vi "Bool array to color.vi"(8 "error in (no error)":errorcluster, 11 "LED Panel":T2) -> (0 "error out":errorcluster, 3 "Calib color":T1)   [LabVIEW 2020]
uses:
  Controls/LED panel ---typedef.ctl
  Controls/Calibration color ---typedef.ctl
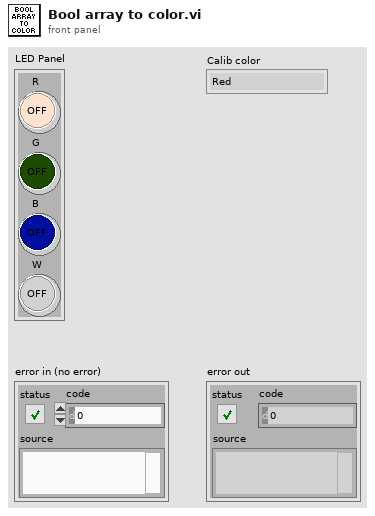
[diagram p1: front panel]
types:
  T1 = typedef "Calibration color ---typedef.ctl" = enum16{"Red", "Green", "Blue", "White", "All", "Reset", "Get"}
  T2 = typedef "LED panel ---typedef.ctl" = cluster{"R":bool, "G":bool, "B":bool, "W":bool}
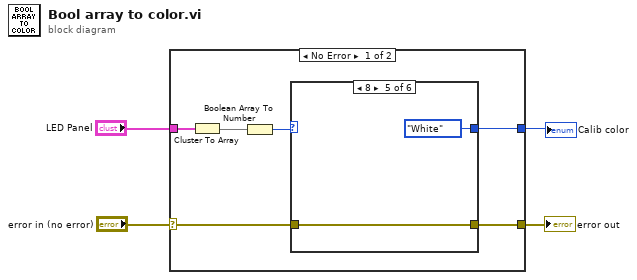
[diagram p0: block diagram]
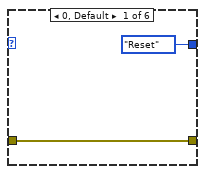
[diagram p2: hidden frame]
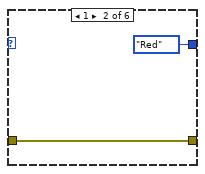
[diagram p3: hidden frame]
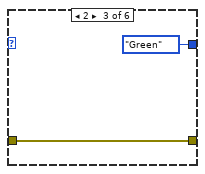
[diagram p4: hidden frame]
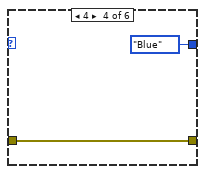
[diagram p5: hidden frame]
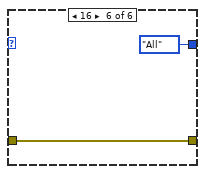
[diagram p6: hidden frame]
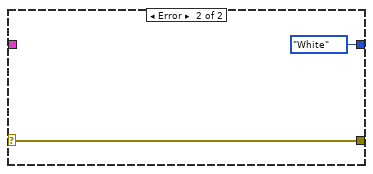
[diagram p7: hidden frame]
diagram:
  n1 = case shown="No Error" "error in (no error)" {
    selector: "error in (no error)" -> [w10 w24]
    tunnel: [w9 w24] -> w3
    tunnel: "LED Panel" -> [w8 _]
    tunnel: [w5 Calibration_color_---typedef."White" ("Calib color")] -> w1
    frame No Error {
      n2 = Cluster To Array(cluster=w8) -> (array=w6:bool[])
      n3 = Boolean Array To Number(Boolean array=w6) -> (number=w7:u32)
      n4 = case shown="8" w7 {
        tunnel: w10 -> [w12 w14 w16 w18 w20 w22]
        tunnel: [w12 w14 w16 w18 w20 w22] -> w9
        tunnel: [Calibration_color_---typedef."Reset" ("Calib color") Calibration_color_---typedef."Red" ("Calib color") Calibration_color_---typedef."Green" ("Calib color") Calibration_color_---typedef."Blue" ("Calib color") Calibration_color_---typedef."White" ("Calib color") Calibration_color_---typedef."All" ("Calib color")] -> w5
        frame 0, Default {
        }
        frame 1 {
        }
        frame 2 {
        }
        frame 4 {
        }
        frame 8 {
        }
        frame 16 {
        }
      }
    }
    frame Error {
    }
  }
  "Calib color" <- w1
  "error out" <- w3
